vi "Limits(DoubleSwitch).vi"(6 "Into Home Limit Is Pos":bool, 8 "Power In":dbl format="%#_13g", 10 "2nd Limit Switch Ref":T1={"DevStatus"={"status"=FALSE, "code"=0, "source"=""}, "DIO Channel"=enum."DIO 1", "CntIndex"=enum."Invalid", "Normally Closed"=FALSE}, 11 "Home Limit Switch Ref":T1={"DevStatus"={"status"=FALSE, "code"=0, "source"=""}, "DIO Channel"=enum."DIO 1", "CntIndex"=enum."Invalid", "Normally Closed"=FALSE}) -> (0 "Power Out":dbl)   [LabVIEW 2018]
uses:
  <vilib>/Rock Robotics/WPI/Switch/WPI_SwitchDevRef.ctl
  <vilib>/Rock Robotics/SystemInterfaces/DIO/FPGA_DIOChannel.ctl
  <vilib>/Rock Robotics/SystemInterfaces/Counter/FPGA_CounterCtrSystemIndex.ctl
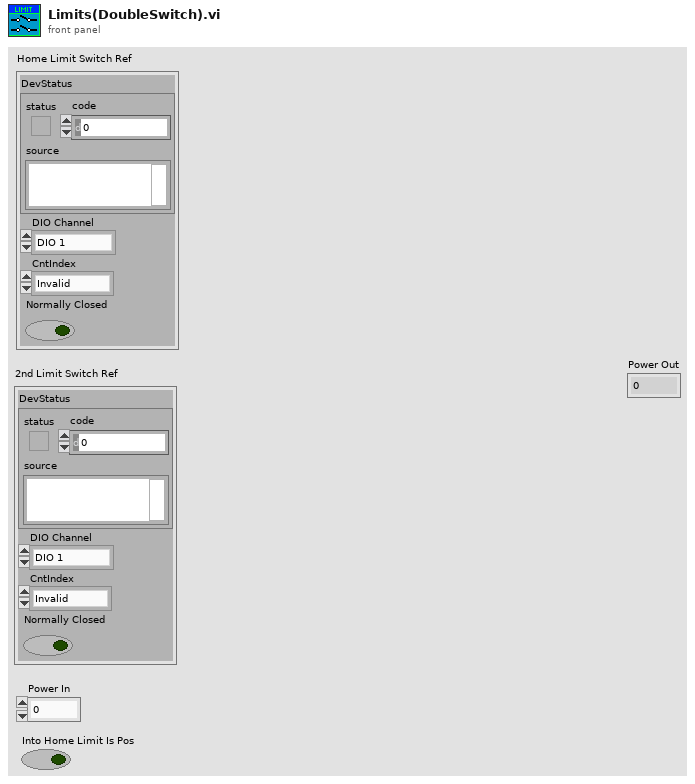
[diagram p1: front panel]
types:
  T1 = typedef "WPI_SwitchDevRef.ctl" = cluster{"DevStatus":errorcluster, "DIO Channel":T2, "CntIndex":T3, "Normally Closed":bool}
  T2 = typedef "FPGA_DIOChannel.ctl" = enum8{"DIO 0", "DIO 1", "DIO 2", "DIO 3", "DIO 4", "DIO 5", "DIO 6", "DIO 7", "DIO 8", "DIO 9", "DIO MXP 0", "DIO MXP 1", "DIO MXP 2", "DIO MXP 3", "DIO MXP 4", "DIO MXP 5", "DIO MXP 6", "DIO MXP 7", "DIO MXP 8", "DIO MXP 9", "DIO MXP 10", "DIO MXP 11", "DIO MXP 12", "DIO MXP 13", "DIO MXP 14", "DIO MXP 15", "SPI Port CS1", "SPI Port CS2", "SPI Port CS3", "SPI Port MISO", "SPI Port MOSI", "Invalid"}
  T3 = typedef "FPGA_CounterCtrSystemIndex.ctl" = enum8{"Ctr 0", "Ctr 1", "Ctr 2", "Ctr 3", "Ctr 4", "Ctr 5", "Ctr 6", "Ctr 7", "Invalid"}
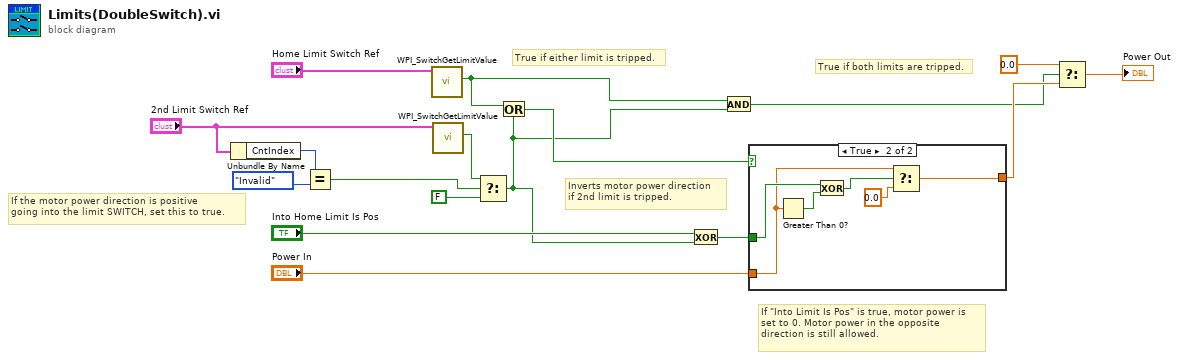
[diagram p0: block diagram]
diagram:
  # "True if both limits are tripped."
  # "If \"Into Limit Is Pos\" is true, motor power is set to 0. Motor power in the opposite direction is still allowed."
  # "True if either limit is tripped."
  # "Inverts motor power direction\nif 2nd limit is tripped."
  # "If the motor power direction is positive\ngoing into the limit SWITCH, set this to true."
  n1 = Unbundle By Name("2nd Limit Switch Ref") -> ("CntIndex"=w10:T3)
  n2 = Equal?(x=w10, y=FPGA_CounterCtrSystemIndex."Invalid" ("CntIndex")) -> (x = y?=w8:bool)
  n3 = call <vilib>:"WPI_SwitchGetLimitValue.vi"("SwitchDevRef"="Home Limit Switch Ref") -> ("Switch Pressed"=w3:bool)  [unwired: 8 in, 2 out]
  n4 = call <vilib>:"WPI_SwitchGetLimitValue.vi"("SwitchDevRef"="2nd Limit Switch Ref") -> ("Switch Pressed"=w11:bool)  [unwired: 8 in, 2 out]
  n5 = Select(t=w11, s=w8, f=FALSE) -> (s? t:f=w2:bool)
  n6 = Or(x=w3, y=w2) -> (x .or. y?=w14:bool)
  n7 = Exclusive Or(1:w2, 2:"Into Home Limit Is Pos") -> (0:w13:bool)
  n8 = And(x=w3, y=w2) -> (x .and. y?=w1:bool)
  n9 = case shown="True" w14 {
    tunnel: [w18 w21] -> w5
    tunnel: w13 -> [_ w20]
    tunnel: "Power In" -> [w18 w19]
    frame False {
    }
    frame True {
      n10 = Greater Than 0?(x=w19) -> (x > 0?=w23:bool)
      n11 = Exclusive Or(1:w23, 2:w20) -> (0:w22:bool)
      n12 = Select(t=w19, s=w22, f=0.0) -> (s? t:f=w21:dbl)
    }
  }
  n13 = Select(t=0.0, s=w1, f=w5) -> (s? t:f=→"Power Out":dbl)
